vi "PQfreeCancel.vi"(8 "error in (no error)":errorcluster, 11 "cancel":u64) -> (0 "error out":errorcluster, 3 "cancel_out":u64)   [LabVIEW 2019, in "libpqlv64.lvlib"]
uses:
  libpqlv64.lvlib
  libpq.dll
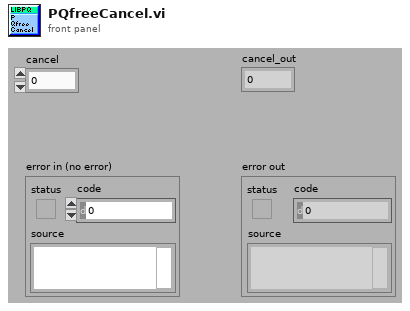
[diagram p1: front panel]
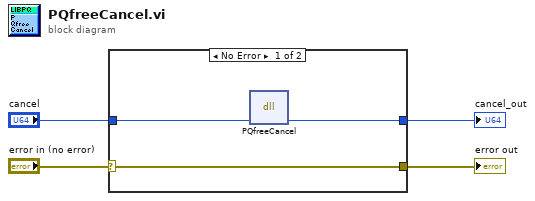
[diagram p0: block diagram]
diagram:
  n1 = case shown="No Error" "error in (no error)" {
    selector: "error in (no error)" -> [w7 w9]
    tunnel: [w7 w9] -> w3
    tunnel: [w6 w8] -> w2
    tunnel: "cancel" -> [w5 w8]
    frame No Error {
      n2 = dll-call lib="libpq.*" fn="PQfreeCancel"("cancel"=w5) -> ("cancel"=w6:u64)  [unwired: 4 in, 2 out]
    }
    frame Error {
    }
  }
  "error out" <- w3
  "cancel_out" <- w2
